vi "Robot.vi"(2 "error in":errorcluster, 3 "Type":enum16{"Mini45", "Joystick"}(ring)=enum."Joystick") -> (0 "error out":errorcluster)   [LabVIEW 2017]
uses:
  <vilib>/Analysis/Matrix/Datatypes/RealMatrix.ctl
  Control/Motor Position.ctl
  Control/Constants.ctl
  Control/Platform Vectors.ctl
  Control/Torque Vector.ctl
  <vilib>/Analysis/baseanly.llb/A x Vector.vi
  <vilib>/Analysis/baseanly.llb/Mean (DBL).vi
  <vilib>/Analysis/baseanly.llb/Real A x B.vi
  <vilib>/DAQmx/read.llb/DAQmx Read (Analog 2D DBL NChan NSamp).vi
  <vilib>/Analysis/_algsub.llb/Vector Norm.vi
  <vilib>/Analysis/_algsub.llb/Real Vector Norm.vi
  <vilib>/Analysis/baseanly.llb/Outer Product.vi
  <vilib>/Analysis/baseanly.llb/Real Outer Product.vi
  <vilib>/robotics/Kinematics/Create Lie Group Matrix.vi
  <vilib>/Analysis/7linalg.llb/Create Special Real Matrix.vi
  <vilib>/Analysis/Matrix/Numeric/Multiply/Multiply.vi
  <vilib>/Analysis/Matrix/Numeric/Multiply/Multiply - RM,R.vi
  <vilib>/Analysis/Matrix/Numeric/Multiply/Multiply - R,RM.vi
  <vilib>/Analysis/Matrix/Numeric/Add/Add.vi
  <vilib>/Analysis/Matrix/Numeric/Add/Add - RM,RM.vi
  <vilib>/Analysis/3filter.llb/Butterworth Filter (DBL).vi
  Global.vi
  <vilib>/Utility/inputDevices.llb/joystickAcquire.vi
  <vilib>/DAQmx/create/channels.llb/DAQmx Create Channel (AI-Voltage-Basic).vi
  <vilib>/DAQmx/configure/timing.llb/DAQmx Timing (Sample Clock).vi
  <vilib>/DAQmx/miscellaneous.llb/DAQmx Fill In Error Info.vi
  <vilib>/Analysis/NI_AALBase.lvlib
  <vilib>/robotics/Kinematics/NI_Kinematics.lvlib
  <vilib>/Analysis/NI_AALPro.lvlib
  <vilib>/Analysis/Matrix/NI_Matrix.lvlib
panel:
  in  "Hz":dbl=100.0 format="%#_13g"
  in  "low cutoff freq: fl":dbl=0.1 format="%0.4f"
  in  "sampling freq: fs":dbl=100.0 format="%0.2f"
  in  "rate":dbl=1000.0 format="%#_13g"
  in  "eta3":dbl=240.0
  in  "eta2":dbl=120.0
  in  "eta1":dbl
  in  "gamma2":dbl=72.0
  in  "gamma1":dbl=90.0
  in  "alpha2":dbl=90.0
  in  "alpha1":dbl=90.0
  in  "radius":dbl=0.1
  in  "Calibration Matrix":T1=[[0.70287, 0.28046, -1.06379, -47.58271, -1.64459, 46.90249], [-0.12905, 55.12684, -1.23322, -27.09022, 0.94146, -27.44249], [69.23154, 1.17633, 67.18151, 0.05352, 69.14468, -0.82584], [0.02366, 0.38743, -1.10802, -0.19684, 1.1351, -0.20033], [1.26658, 0.02633, -0.60731, 0.32903, -0.6386, -0.32248], [0.02624, -0.70869, -0.00313, -0.69424, -0.02408, -0.68399]]
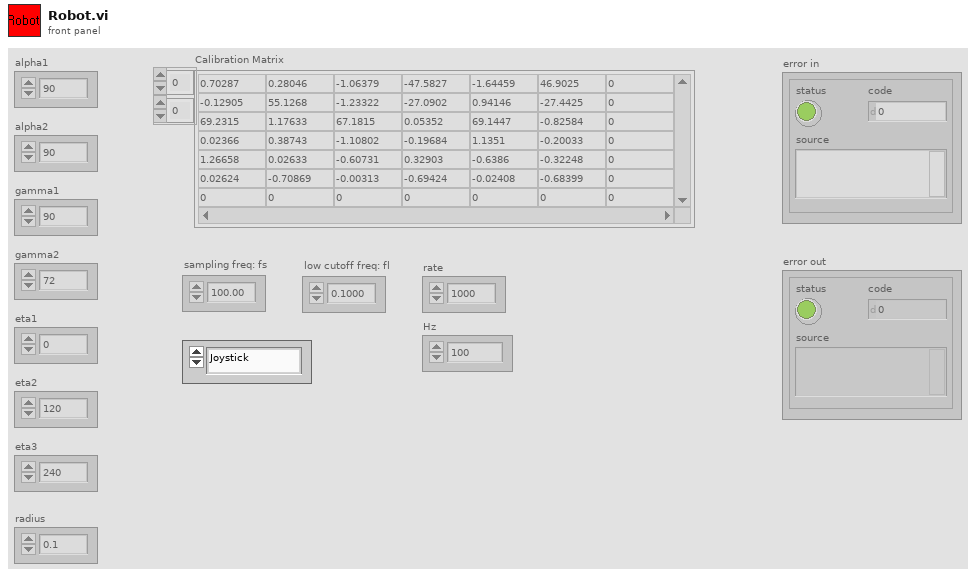
[diagram p1: front panel]
types:
  T1 = typedef "NI_Matrix.lvlib/RealMatrix.ctl" = dbl[][]
  T2 = typedef "Motor Position.ctl" = cluster{"theta1":dbl, "theta2":dbl, "theta3":dbl}
  T3 = typedef "Platform Vectors.ctl" = cluster{"v1":dbl[], "v2":dbl[], "v3":dbl[]}
  T4 = typedef "Constants.ctl" = cluster{"alpha1":dbl, "alpha2":dbl, "beta1":dbl, "beta2":dbl, "gamma1":dbl, "gamma2":dbl, "eta1":dbl, "eta2":dbl, "eta3":dbl}
  T5 = typedef "Torque Vector.ctl" = cluster{"Tx":dbl, "Ty":dbl, "Tz":dbl}
  T6 = cluster{"X axis":i32, "Y axis":i32, "Z axis":i32, "X axis rotation":i32, "Y axis rotation":i32, "Z axis rotation":i32, "U axis":i32, "V axis":i32}
  T7 = typedef "Damping.ctl" = cluster{"bx":dbl, "by":dbl, "bz":dbl}
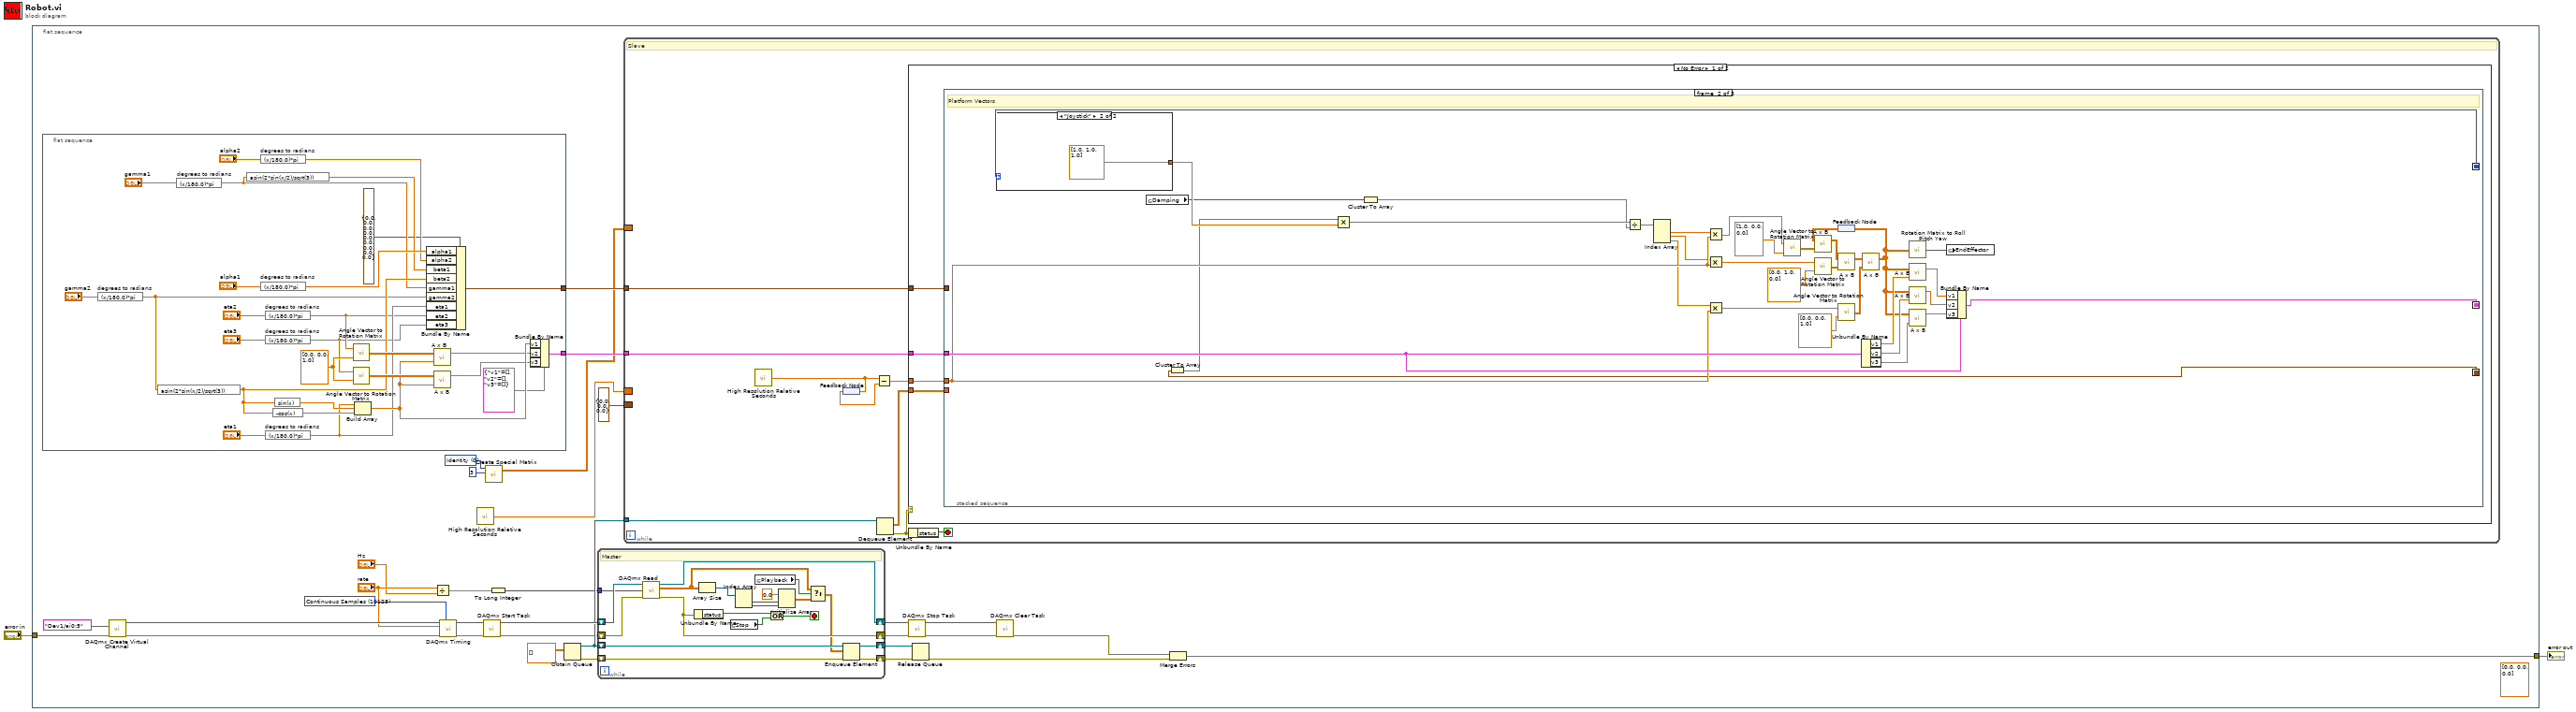
[diagram p0: block diagram]
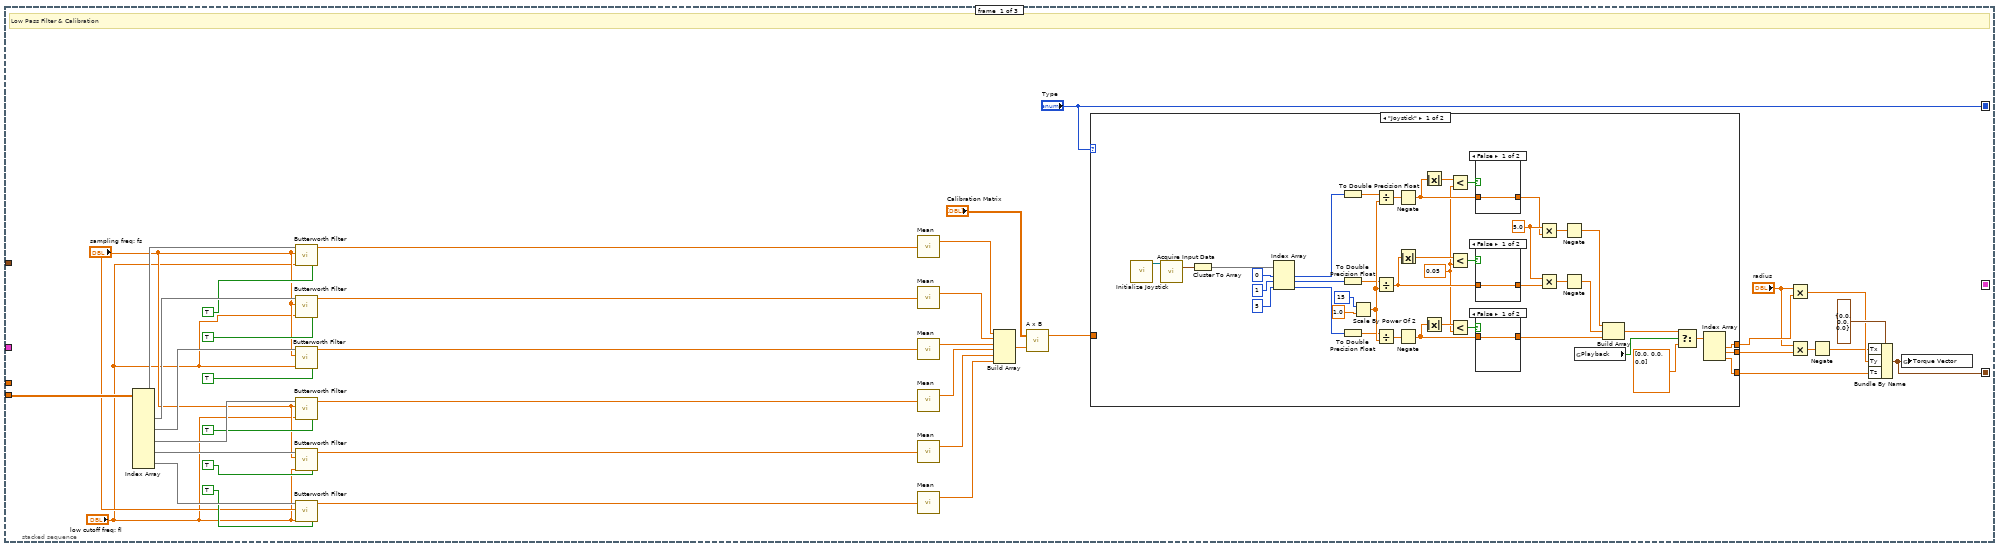
[diagram p2: hidden frame]
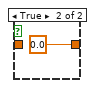
[diagram p3: hidden frame]
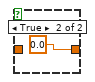
[diagram p4: hidden frame]
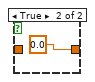
[diagram p5: hidden frame]
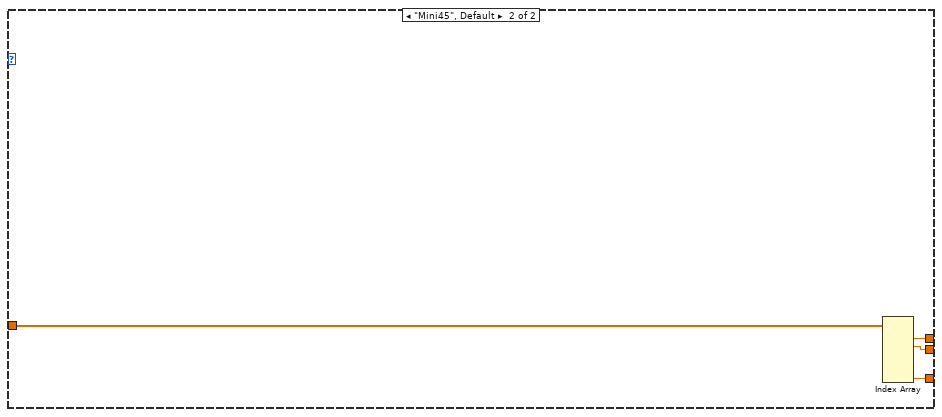
[diagram p6: hidden frame]
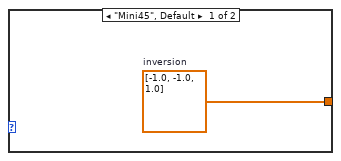
[diagram p7: hidden frame]
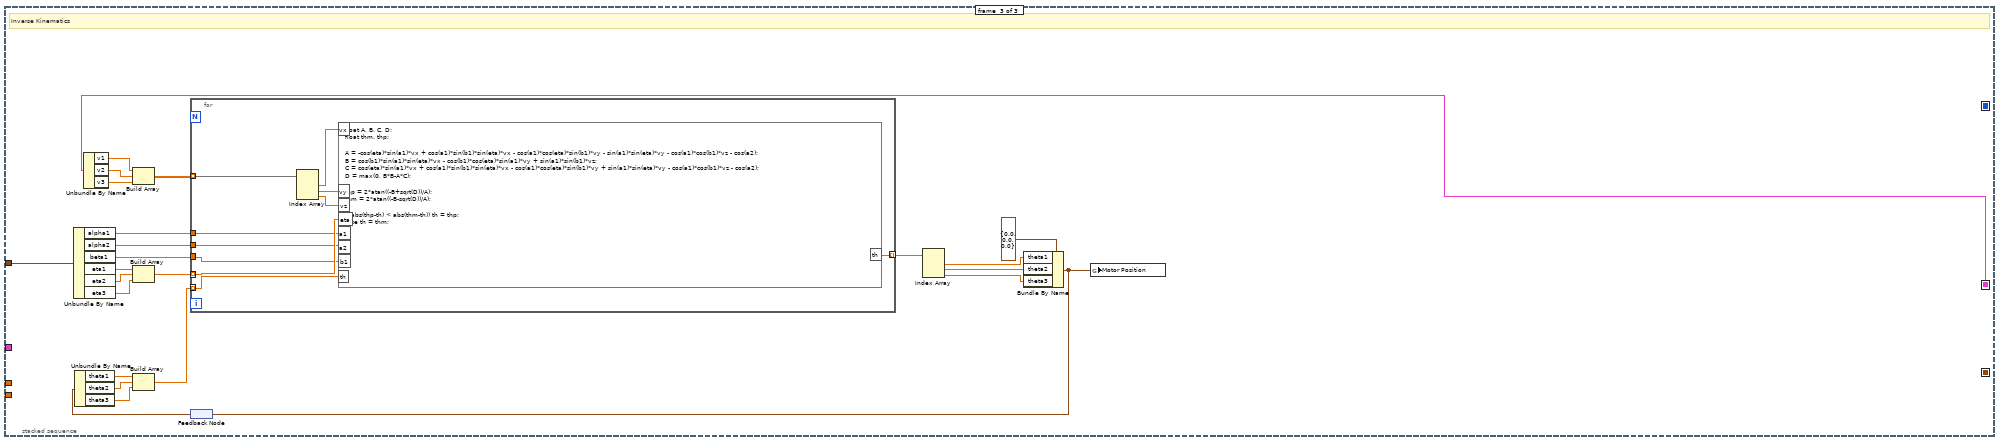
[diagram p8: hidden frame]
diagram:
  n1 = flat-sequence {
    tunnel: "error in" -> [w5]
    tunnel: [w3] -> w1
    frame #0 {
      w16 = 0 items=["Identity", "Diagonal", "Toeplitz", "Vandermonde", "Companion", "Hankel", "Hadamard", "Wilkinson", "Hilbert", "Inverse Hilbert", "Rosser", "Pascal"] ("matrix type")
      (unwired) dbl[] [0.0, 0.0, 0.0]
      w22 = 10123 items=["Finite Samples"=10178, "Continuous Samples"=10123, "Hardware Timed Single Point"=12522] ("sample mode")
      n2 = flat-sequence {
        tunnel: [w62] -> w34
        tunnel: [w61] -> w33
        frame #0 {
          w49 = dbl[] [0.0, 0.0, 1.0] ("vector")
          n3 = expression code="(x/180.0)*pi" "degrees to radians"("gamma2") -> (w43:dbl)
          n4 = expression code="asin(2*sin(x/2)/sqrt(3))"(w43) -> (w45:dbl)
          n5 = expression code="(x/180.0)*pi" "degrees to radians"("gamma1") -> (w44:dbl)
          n6 = expression code="asin(2*sin(x/2)/sqrt(3))"(w44) -> (w56:dbl)
          n7 = expression code="(x/180.0)*pi" "degrees to radians"("alpha2") -> (w57:dbl)
          n8 = expression code="(x/180.0)*pi" "degrees to radians"("alpha1") -> (w59:dbl)
          n9 = expression code="(x/180.0)*pi" "degrees to radians"("eta2") -> (w38:dbl)
          n10 = expression code="(x/180.0)*pi" "degrees to radians"("eta3") -> (w37:dbl)
          n11 = expression code="(x/180.0)*pi" "degrees to radians"("eta1") -> (w39:dbl)
          n12 = expression code="-cos(x)"(w45) -> (w51:dbl)
          n13 = expression code="sin(x)"(w45) -> (w50:dbl)
          n14 = call <vilib>:"Angle Vector to Rotation Matrix.vi"("vector"=w49, "angle"=w38) -> ("rotation matrix"=w52:T1)
          n15 = call <vilib>:"Angle Vector to Rotation Matrix.vi"("vector"=w49, "angle"=w37) -> ("rotation matrix"=w53:T1)
          n16 = Build Array(w39, w50, w51) -> (w48:dbl[])
          n17 = Bundle By Name(cluster=T4 {"alpha1"=0.0, "alpha2"=0.0, "beta1"=0.0, "beta2"=0.0, "gamma1"=0.0, "gamma2"=0.0, "eta1"=0.0, "eta2"=0.0, "eta3"=0.0} ("Constants"), "alpha1"=w59, "alpha2"=w57, "beta1"=w56, "beta2"=w45, "gamma1"=w44, "gamma2"=w43, "eta1"=w39, "eta2"=w38, "eta3"=w37) -> (w61:T4)
          n18 = call-poly <vilib>:"A x B.vi"("Vector"=w48, "A"=w52) -> ("A x Vector"=w47:dbl[])  [unwired: 1 out]
          n19 = call-poly <vilib>:"A x B.vi"("Vector"=w48, "A"=w53) -> ("A x Vector"=w46:dbl[])  [unwired: 1 out]
          n20 = Bundle By Name(cluster=T3 {"v1"=[], "v2"=[], "v3"=[]} ("Platform Vectors"), "v1"=w48, "v2"=w47, "v3"=w46) -> (w62:T3)
        }
      }
      n21 = call-poly <vilib>:"DAQmx Create Virtual Channel.vi"("physical channels"=tag "Dev1/ai0:5", "error in"=w5) -> ("task out"=w31:refnum<k21>, "error out"=w30:errorcluster)  [unwired: 12 in]
      n22 = Divide(x="rate", y="Hz") -> (x/y=w6:dbl)
      n23 = call-poly <vilib>:"DAQmx Timing.vi"("task/channels in"=w31, "sample mode"=w22, "rate"="rate", "error in"=w30) -> ("task out"=w28:refnum<k21>, "error out"=w29:errorcluster)  [unwired: 10 in]
      n24 = call <vilib>:"High Resolution Relative Seconds.vi"() -> ("relative seconds"=w7:dbl)
      n25 = call <vilib>:"DAQmx Start Task.vi"("task/channels in"=w28, "error in"=w29) -> ("task out"=w27:refnum<k21>, "error out"=w4:errorcluster)  [unwired: 12 in]
      n26 = call-poly <vilib>:"Create Special Matrix.vi"("matrix type"=w16, "matrix size"=3) -> ("Special Matrix"=w14:T1)  [unwired: 3 in, 1 out]
      n27 = To Long Integer(number=w6) -> (32bit integer=w9:i32)
      n28 = Obtain Queue(element data type=dbl[][] [] ("data")) -> (queue out=w12:refnum<queue>, error out=w21:errorcluster)  [unwired: 4 in, 1 out]
      n29 = while {
        shift-right: [w252] -> w19
        shift-left: w12 -> [w253]
        shift-right: [w249] -> w18
        shift-left: w21 -> [w251]
        shift-right: [w256] -> w26
        shift-left: w27 -> [w257]
        shift-right: [w254] -> w24
        shift-left: w4 -> [w255]
        tunnel: w9 -> [w247]
        stop <- w248 stop-if-true
        # "Master"
        n30 = call-poly <vilib>:"DAQmx Read.vi"("task/channels in"=w257, "number of samples per channel"=w247, "error in"=w255) -> ("task out"=w256:refnum<k21>, "data"=w243:dbl[][], "error out"=w254:errorcluster)  [unwired: 10 in]
        n31 = Unbundle By Name(w254) -> ("status"=w250:bool)
        n32 = Array Size(array=w243) -> (size(s)=w242:i32[])
        n33 = global read "Global.vi" "Stop"() -> (w246:bool)
        n34 = Index Array(array=w242) -> (element #1=w241:i32, element #2=w240:i32)  [unwired: 2 in]
        n35 = global read "Global.vi" "Playback"() -> (w245:bool)
        n36 = Compound Arithmetic op=OR(w250, w246) -> (w248:bool)
        n37 = Initialize Array(0.0 ("element"), w241, w240) -> (w238:dbl[][])
        n38 = Select(t=w243, s=w245, f=w238) -> (s? t:f=w244:dbl[][])
        n39 = Enqueue Element(queue=w253, element=w244, error in (no error)=w251) -> (queue out=w252:refnum<queue>, error out=w249:errorcluster)  [unwired: 1 in, 1 out]
      }
      n40 = while {
        tunnel: w12 -> [w71]
        border: w14 -> [_]
        tunnel: w33 -> [w69]
        border: T2 {"theta1"=0.0, "theta2"=0.0, "theta3"=0.0} ("Motor Position") -> [_]
        border: w7 -> [_]
        tunnel: w34 -> [w70]
        stop <- w63 stop-if-true
        # "Slave"
        n41 = call <vilib>:"High Resolution Relative Seconds.vi"() -> ("relative seconds"=w65:dbl)
        n42 = feedback-in #1(w65) -> ()
        n43 = feedback #1() -> (w66:dbl)
        n44 = Subtract(x=w65, y=w66) -> (x-y=w64:dbl)
        n45 = Dequeue Element(queue=w71) -> (element=w67:dbl[][], error out=w68:errorcluster)  [unwired: 2 in, 2 out]
        n46 = case shown="No Error" w68 {
          tunnel: w70 -> [w75 _]
          tunnel: w69 -> [w74 _]
          tunnel: w67 -> [w73 _]
          tunnel: w64 -> [w72 _]
          frame No Error {
            n47 = stacked-sequence {
              seq-local: [w80 _ _] -> [_ w170 _]
              seq-local: [_ w185 _] -> [_ _ w206]
              seq-local: ["Type" _ _] -> [_ w168 _]
              tunnel: w75 -> [_ w187 _]
              tunnel: w74 -> [_ _ w223]
              tunnel: w72 -> [_ w184 _]
              tunnel: w73 -> [w91 _ _]
              frame #0 {
                # "Low Pass Filter & Calibration"
                n48 = Index Array(array=w91) -> (element #1=w102:dbl[], element #2=w101:dbl[], element #3=w100:dbl[], element #4=w99:dbl[], element #5=w98:dbl[], element #6=w97:dbl[])  [unwired: 12 in]
                n49 = call-poly <vilib>:"Butterworth Filter.vi"("init/cont (init:F)"=TRUE, "low cutoff freq: fl"="low cutoff freq: fl", "sampling freq: fs"="sampling freq: fs", "X"=w102) -> ("Filtered X"=w103:dbl[])  [unwired: 4 in, 1 out]
                n50 = call-poly <vilib>:"Butterworth Filter.vi"("init/cont (init:F)"=TRUE, "low cutoff freq: fl"="low cutoff freq: fl", "sampling freq: fs"="sampling freq: fs", "X"=w101) -> ("Filtered X"=w105:dbl[])  [unwired: 4 in, 1 out]
                n51 = call-poly <vilib>:"Butterworth Filter.vi"("init/cont (init:F)"=TRUE, "low cutoff freq: fl"="low cutoff freq: fl", "sampling freq: fs"="sampling freq: fs", "X"=w100) -> ("Filtered X"=w107:dbl[])  [unwired: 4 in, 1 out]
                n52 = call-poly <vilib>:"Butterworth Filter.vi"("init/cont (init:F)"=TRUE, "low cutoff freq: fl"="low cutoff freq: fl", "sampling freq: fs"="sampling freq: fs", "X"=w99) -> ("Filtered X"=w108:dbl[])  [unwired: 4 in, 1 out]
                n53 = call-poly <vilib>:"Butterworth Filter.vi"("init/cont (init:F)"=TRUE, "low cutoff freq: fl"="low cutoff freq: fl", "sampling freq: fs"="sampling freq: fs", "X"=w98) -> ("Filtered X"=w109:dbl[])  [unwired: 4 in, 1 out]
                n54 = call-poly <vilib>:"Butterworth Filter.vi"("init/cont (init:F)"=TRUE, "low cutoff freq: fl"="low cutoff freq: fl", "sampling freq: fs"="sampling freq: fs", "X"=w97) -> ("Filtered X"=w113:dbl[])  [unwired: 4 in, 1 out]
                n55 = call-poly <vilib>:"Mean.vi"("X"=w103) -> ("mean"=w104:dbl)  [unwired: 1 out]
                n56 = call-poly <vilib>:"Mean.vi"("X"=w105) -> ("mean"=w106:dbl)  [unwired: 1 out]
                n57 = call-poly <vilib>:"Mean.vi"("X"=w107) -> ("mean"=w110:dbl)  [unwired: 1 out]
                n58 = call-poly <vilib>:"Mean.vi"("X"=w108) -> ("mean"=w111:dbl)  [unwired: 1 out]
                n59 = call-poly <vilib>:"Mean.vi"("X"=w109) -> ("mean"=w112:dbl)  [unwired: 1 out]
                n60 = call-poly <vilib>:"Mean.vi"("X"=w113) -> ("mean"=w114:dbl)  [unwired: 1 out]
                n61 = Build Array(w104, w106, w110, w111, w112, w114) -> (w89:dbl[])
                n62 = call-poly <vilib>:"A x B.vi"("Vector"=w89, "A"="Calibration Matrix") -> ("A x Vector"=w86:dbl[])  [unwired: 1 out]
                n63 = case shown="\"Joystick\"" "Type" {
                  tunnel: w86 -> [_ w167]
                  tunnel: [w123 w166] -> w83
                  tunnel: [w122 w165] -> w81
                  tunnel: [w121 w164] -> w85
                  frame "Joystick" {
                    w130 = 5.0 ("element")
                    w137 = 0.05 ("y")
                    n64 = call <vilib>:"Initialize Joystick.vi"() -> ("device ID"=w150:refnum<k1>)  [unwired: 10 in, 1 out]
                    n65 = call-poly <vilib>:"Acquire Input Data.vi"("device ID"=w150) -> ("axis info"=w157:T6)  [unwired: 14 in, 4 out]
                    n66 = Cluster To Array(cluster=w157) -> (array=w153:i32[])
                    n67 = Index Array(array=w153, index #1=0 ("index"), index #2=1 ("index"), index #3=5 ("index")) -> (element #1=w136:i32, element #2=w134:i32, element #3=w132:i32)
                    n68 = To Double Precision Float(number=w136) -> (double precision float=w135:dbl)
                    n69 = To Double Precision Float(number=w134) -> (double precision float=w133:dbl)
                    n70 = To Double Precision Float(number=w132) -> (double precision float=w131:dbl)
                    n71 = Scale By Power Of 2(n=i16 15, x=1.0) -> (x*2^n=w145:dbl)
                    n72 = Divide(x=w135, y=w145) -> (x/y=w149:dbl)
                    n73 = Divide(x=w133, y=w145) -> (x/y=w140:dbl)
                    n74 = Divide(x=w131, y=w145) -> (x/y=w138:dbl)
                    n75 = Negate(x=w149) -> (-x=w141:dbl)
                    n76 = Absolute Value(x=w140) -> (abs(x)=w147:dbl)
                    n77 = Negate(x=w138) -> (-x=w139:dbl)
                    n78 = Absolute Value(x=w141) -> (abs(x)=w148:dbl)
                    n79 = Absolute Value(x=w139) -> (abs(x)=w146:dbl)
                    n80 = Less?(x=w148, y=w137) -> (x < y?=w144:bool)
                    n81 = Less?(x=w147, y=w137) -> (x < y?=w143:bool)
                    n82 = Less?(x=w146, y=w137) -> (x < y?=w142:bool)
                    n83 = case shown="False" w144 {
                      tunnel: [w162 0.0] -> w129
                      tunnel: w141 -> [w162 _]
                      frame False {
                      }
                      frame True {
                      }
                    }
                    n84 = case shown="False" w143 {
                      tunnel: [w160 0.0] -> w128
                      tunnel: w140 -> [w160 _]
                      frame False {
                      }
                      frame True {
                      }
                    }
                    n85 = case shown="False" w142 {
                      tunnel: [w158 0.0] -> w126
                      tunnel: w139 -> [w158 _]
                      frame False {
                      }
                      frame True {
                      }
                    }
                    n86 = Multiply(x=w130, y=w129) -> (x*y=w119:dbl)
                    n87 = Multiply(x=w130, y=w128) -> (x*y=w117:dbl)
                    n88 = Negate(x=w119) -> (-x=w118:dbl)
                    n89 = Negate(x=w117) -> (-x=w116:dbl)
                    n90 = global read "Global.vi" "Playback"() -> (w127:bool)
                    n91 = Build Array(w118, w116, w126) -> (w125:dbl[])
                    n92 = Select(t=w125, s=w127, f=dbl[] [0.0, 0.0, 0.0]) -> (s? t:f=w124:dbl[])
                    n93 = Index Array(array=w124) -> (element #1=w123:dbl, element #2=w122:dbl, element #3=w121:dbl)  [unwired: 3 in]
                  }
                  frame "Mini45", Default {
                    n94 = Index Array(array=w167) -> (element #1=w166:dbl, element #2=w165:dbl, element #6=w164:dbl)  [unwired: 6 in, 3 out]
                  }
                }
                n95 = Multiply(x="radius", y=w83) -> (x*y=w79:dbl)
                n96 = Multiply(x="radius", y=w81) -> (x*y=w78:dbl)
                n97 = Negate(x=w78) -> (-x=w77:dbl)
                n98 = Bundle By Name(cluster=T5 {"Tx"=0.0, "Ty"=0.0, "Tz"=0.0} ("Torque Vector"), "Tx"=w77, "Ty"=w79, "Tz"=w85) -> (w80:T5)
                n99 = global write "Global.vi" "Torque Vector"(w80) -> ()
              }
              frame #1 {
                # "Platform Vectors"
                n100 = case shown="\"Joystick\"" w168 {
                  tunnel: [w202 dbl[] [1.0, 1.0, 1.0]] -> w186
                  frame "Mini45", Default {
                    w202 = dbl[] [-1.0, -1.0, 1.0]  # inversion
                  }
                  frame "Joystick" {
                  }
                }
                n101 = global read "Global.vi" "Damping"() -> (w177:T7)
                n102 = Cluster To Array(cluster=w170) -> (array=w169:dbl[])
                n103 = Multiply(x=w169, y=w186) -> (x*y=w178:dbl[])
                n104 = Cluster To Array(cluster=w177) -> (array=w176:dbl[])
                n105 = Divide(x=w178, y=w176) -> (x/y=w175:dbl[])
                n106 = Index Array(array=w175) -> (element #1=w174:dbl, element #2=w173:dbl, element #3=w172:dbl)  [unwired: 3 in]
                n107 = Multiply(x=w174, y=w184) -> (x*y=w201:dbl)
                n108 = Multiply(x=w173, y=w184) -> (x*y=w200:dbl)
                n109 = Multiply(x=w172, y=w184) -> (x*y=w183:dbl)
                n110 = call <vilib>:"Angle Vector to Rotation Matrix.vi"("vector"=dbl[] [1.0, 0.0, 0.0], "angle"=w201) -> ("rotation matrix"=w196:T1)
                n111 = call <vilib>:"Angle Vector to Rotation Matrix.vi"("vector"=dbl[] [0.0, 1.0, 0.0], "angle"=w200) -> ("rotation matrix"=w194:T1)
                n112 = feedback #2() -> (w191:T1)
                n113 = call-poly <vilib>:"A x B.vi"("B"=w196, "A"=w191) -> ("A x B"=w195:T1)  [unwired: 1 out]
                n114 = call-poly <vilib>:"A x B.vi"("B"=w194, "A"=w195) -> ("A x B"=w193:T1)  [unwired: 1 out]
                n115 = call <vilib>:"Angle Vector to Rotation Matrix.vi"("vector"=dbl[] [0.0, 0.0, 1.0], "angle"=w183) -> ("rotation matrix"=w192:T1)
                n116 = Unbundle By Name(w187) -> ("v1"=w190:dbl[], "v2"=w189:dbl[], "v3"=w188:dbl[])
                n117 = call-poly <vilib>:"A x B.vi"("B"=w192, "A"=w193) -> ("A x B"=w179:T1)  [unwired: 1 out]
                n118 = feedback-in #2(w179) -> ()
                n119 = call <vilib>:"Rotation Matrix to Roll Pitch Yaw.vi"("rotation matrix"=w179) -> ("angles"=w171:cluster{"roll":dbl, "pitch":dbl, "yaw":dbl})
                n120 = call-poly <vilib>:"A x B.vi"("Vector"=w190, "A"=w179) -> ("A x Vector"=w182:dbl[])  [unwired: 1 out]
                n121 = call-poly <vilib>:"A x B.vi"("Vector"=w189, "A"=w179) -> ("A x Vector"=w181:dbl[])  [unwired: 1 out]
                n122 = call-poly <vilib>:"A x B.vi"("Vector"=w188, "A"=w179) -> ("A x Vector"=w180:dbl[])  [unwired: 1 out]
                n123 = global write "Global.vi" "EndEffector"(w171) -> ()
                n124 = Bundle By Name(cluster=w187, "v1"=w182, "v2"=w181, "v3"=w180) -> (w185:T3)
              }
              frame #2 {
                # "Inverse Kinematics"
                n125 = Unbundle By Name(w223) -> ("alpha1"=w218:dbl, "alpha2"=w217:dbl, "beta1"=w216:dbl, "eta1"=w222:dbl, "eta2"=w221:dbl, "eta3"=w220:dbl)
                n126 = Unbundle By Name(w206) -> ("v1"=w227:dbl[], "v2"=w226:dbl[], "v3"=w225:dbl[])
                n127 = Build Array(w227, w226, w225) -> (w224:dbl[][])
                n128 = Build Array(w222, w221, w220) -> (w219:dbl[])
                n129 = feedback #3() -> (w211:T2)
                n130 = Unbundle By Name(w211) -> ("theta1"=w210:dbl, "theta2"=w209:dbl, "theta3"=w208:dbl)
                n131 = Build Array(w210, w209, w208) -> (w207:dbl[])
                n132 = for {
                  tunnel: w224 -> [w237] mode=indexing
                  tunnel: w219 -> [w233] mode=indexing
                  tunnel: w218 -> [w232]
                  tunnel: w217 -> [w231]
                  tunnel: w216 -> [w230]
                  tunnel: [w229] -> w215 mode=indexing
                  tunnel: w207 -> [w228] mode=indexing
                  n133 = Index Array(array=w237) -> (element #1=w236:dbl, element #2=w235:dbl, element #3=w234:dbl)  [unwired: 3 in]
                  n134 = formula code="float A, B, C, D;\nfloat thm, thp;\n\nA = -cos(eta)*sin(a1)*vx + cos(a1)*sin(b1)*sin(eta)*vx - cos(a1)*cos(eta)*sin(b1)*vy - sin(a1)*sin(eta)*vy - cos(a1)*cos(b1)*vz - cos(a2);\nB = cos(b1)*sin(a1)*sin(eta)*vx - cos(b1)*cos(eta)*sin(a1)*vy + sin(a1)*sin(b1)*vz;\nC = cos(eta)*sin(a1)*vx + cos(a1)*sin(b1)*sin(eta)*vx - cos(a1)*cos(eta)*sin(b1)*vy + sin(a1)*sin(eta)*vy - cos(a1)*cos(b1)*vz - cos(a2);\nD = max(0, B*B-A*C);\n\nthp = 2*atan((-B+sqrt(D))/A); \nthm = 2*atan((-B-sqrt(D))/A); \n\nif(abs(thp-th) < abs(thm-th)) th = thp;\nelse th = thm;"("vx"=w236, "vy"=w235, "vz"=w234, "eta"=w233, "a1"=w232, "b1"=w230, "a2"=w231, "th"=w228) -> ("th"=w229:dbl)
                }
                n135 = Index Array(array=w215) -> (element #1=w214:dbl, element #2=w213:dbl, element #3=w212:dbl)  [unwired: 3 in]
                n136 = Bundle By Name(cluster=T2 {"theta1"=0.0, "theta2"=0.0, "theta3"=0.0} ("Motor Position"), "theta1"=w214, "theta2"=w213, "theta3"=w212) -> (w204:T2)
                n137 = feedback-in #3(w204) -> ()
                n138 = global write "Global.vi" "Motor Position"(w204) -> ()
              }
            }
          }
          frame Error {
          }
        }
        n139 = Unbundle By Name(w68) -> ("status"=w63:bool)
      }
      n140 = call <vilib>:"DAQmx Stop Task.vi"("task/channels in"=w26, "error in"=w24) -> ("task out"=w25:refnum<k21>, "error out"=w23:errorcluster)  [unwired: 12 in]
      n141 = Release Queue(queue=w19, error in (no error)=w18) -> (error out=w17:errorcluster)  [unwired: 1 in, 2 out]
      n142 = call <vilib>:"DAQmx Clear Task.vi"("task in"=w25, "error in"=w23) -> ("error out"=w20:errorcluster)  [unwired: 13 in]
      n143 = Merge Errors(w20, w17) -> (w3:errorcluster)
    }
  }
  "error out" <- w1
